vi "Resampling for Power Measurement.vi"(7 "reset? (F)":bool, 8 "error in (no error)":errorcluster, 9 "samples per cycle (192)":u16=192, 10 "trigger information":T2={"trigger times [s]"=[], "triggers per cycle"=2}, 11 "data in":waveform(dbl)[](array[waveform])) -> (0 "error out":errorcluster, 3 "resampled data":T1[](array[typedef]) {"resampled signal" format="%.2f"; "times [s]" format="%.2f"})   [LabVIEW 2014, in "NI_EP_Power Measurement.lvlib"]
doc: "Resamples even-time-spaced voltage and current signals into even-angle-spaced signals for harmonic analysis, according to the trigger times that you specify."
uses:
  <vilib>/addons/Electrical Power/Power Measurement/NI_EP_Power Measurement.lvlib
  <vilib>/addons/Electrical Power/Power Measurement/subVIs/ep_Resampled Data.ctl
  <vilib>/Analysis/2dsp.llb/Resample (constant to variable, multi-channel).vi
  <vilib>/Analysis/NI_AALPro.lvlib
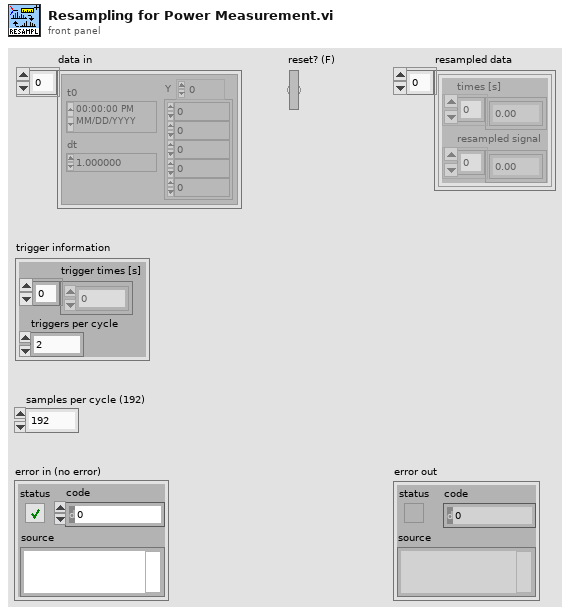
[diagram p1: front panel]
types:
  T1 = typedef "NI_EP_Power Measurement.lvlib/ep_Resampled Data.ctl" = cluster{"times [s]":dbl[], "resampled signal":dbl[]}
  T2 = cluster{"trigger times [s]":dbl[], "triggers per cycle":u8}
  T3 = cluster{"alias rejection (dB)":dbl, "normalized bandwidth":dbl}
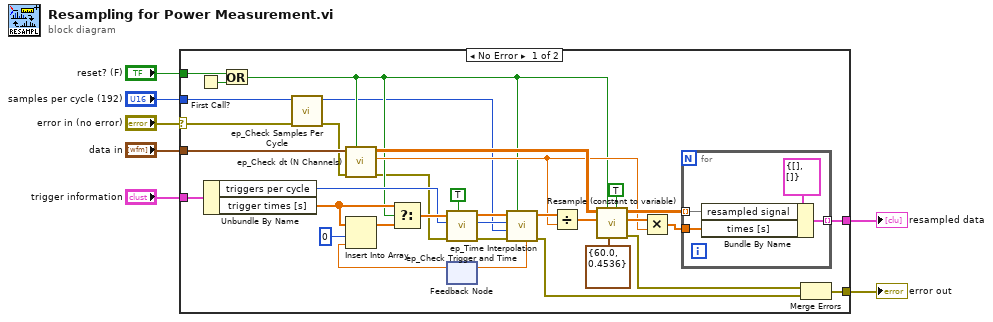
[diagram p0: block diagram]
diagram:
  n1 = case shown="No Error" "error in (no error)" {
    selector: "error in (no error)" -> [w11 w46]
    tunnel: "trigger information" -> [w29 _]
    tunnel: "samples per cycle (192)" -> [w16 _]
    tunnel: "reset? (F)" -> [w40 _]
    tunnel: "data in" -> [w20 _]
    tunnel: [w30 _] -> w3
    tunnel: [w10 w46] -> w4
    frame No Error {
      n2 = First Call?() -> (First Call?: T/F=w41:bool)
      n3 = Unbundle By Name(w29) -> ("triggers per cycle"=w22:u8, "trigger times [s]"=w37:dbl[])
      n4 = Or(x=w40, y=w41) -> (x .or. y?=w15:bool)
      n5 = call <vilib>:"ep_Check Samples Per Cycle.vi"("error in (no error)"=w11, "samples per cycle"=w16) -> ("error out"=w13:errorcluster, "dup samples per cycle"=w14:u16)  [unwired: 8 in]
      n6 = call <vilib>:"ep_Check dt (N Channels).vi"("reset? (F)"=w15, "error in (no error)"=w13, "waveforms"=w20) -> ("error out"=w12:errorcluster, "dt"=w18:dbl, "signals"=w19:dbl[][])  [unwired: 4 in, 2 out]
      n7 = feedback #1() -> (w39:dbl)  [unwired: 1 in]
      n8 = Insert Into Array(array=w37, index=0, new element=w39) -> (w38:dbl[])
      n9 = Select(t=w37, s=w15, f=w38) -> (s? t:f=w28:dbl[])
      n10 = call <vilib>:"ep_Check Trigger and Time.vi"("trigger? (F)"=TRUE ("trigger? (T)"), "error in (no error)"=w12, "triggers per cycle"=w22, "trigger/positions [s]"=w28) -> ("error out"=w26:errorcluster, "dup triggers per cycle"=w24:u8, "dup trigger/positions [s]"=w25:dbl[])  [unwired: 5 in]
      n11 = call <vilib>:"ep_Time Interpolation.vi"("reset? (F)"=w15, "error in (no error)"=w26, "samples per cycle"=w14, "triggers per cycle"=w24, "trigger positions [s]"=w25) -> ("error out"=w8:errorcluster, "time index"=w21:dbl[], "last position [s]"=w23:dbl)  [unwired: 4 in]
      n12 = feedback-in #1(w23) -> ()
      n13 = Divide(x=w21, y=w18) -> (x/y=w33:dbl[])
      n14 = call-poly <vilib>:"Resample (constant to variable).vi"("anti-aliasing?"=TRUE, "FIR filter specifications"=T3 {"alias rejection (dB)"=60.0, "normalized bandwidth"=0.4536}, "reset?"=w15, "Time"=w33, "X"=w19) -> ("error out"=w9:errorcluster, "Time Stamps"=w31:dbl[], "Y"=w34:dbl[][])  [unwired: 4 in]
      n15 = Multiply(x=w31, y=w18) -> (x*y=w32:dbl[])
      n16 = for {
        tunnel: w34 -> [w45] mode=indexing
        tunnel: w32 -> [w44]
        tunnel: [w43] -> w30 mode=indexing
        n17 = Bundle By Name(cluster=T1 {"times [s]"=[], "resampled signal"=[]} ("resampled data"), "resampled signal"=w45, "times [s]"=w44) -> (w43:T1)
      }
      n18 = Merge Errors(w9, w8) -> (w10:errorcluster)
    }
    frame Error {
    }
  }
  "error out" <- w4
  "resampled data" <- w3
